vi "Send.vi"(6 "Timeout":T1={"mode"=enum."Relative", "deadline (ms)"=30000}, 7 "priority":bool, 8 "error in (no error)":errorcluster, 9 "path":string, 10 "session in":refnum<class "Session.lvclass">, 11 "NI_SFTP.lvlib:statvfs_openssh.com.lvclass":refnum<class "statvfs_openssh.com.lvclass">) -> (0 "error out":errorcluster, 1 "request id":u32, 2 "session out":refnum<class "Session.lvclass">, 3 "NI_SFTP.lvlib:statvfs_openssh.com.lvclass 2":refnum<class "statvfs_openssh.com.lvclass">)   [LabVIEW 2020, in "NI_SFTP.lvlib" / "statvfs_openssh.com.lvclass"]
uses:
  <vilib>/net/SFTP/API/Support/Command/statvfs_openssh.com/statvfs_openssh.com.lvclass
  <vilib>/net/SFTP/Session/Session.lvclass
  <vilib>/Utility/Deadline/Deadline.ctl
  <vilib>/Utility/Deadline/Mode.ctl
  <vilib>/net/SFTP/API/Support/Command/SSH_FXP_EXTENDED/Input.ctl
  <vilib>/net/SFTP/Low Level Connection/Serialize Byte Array.vi
  <vilib>/net/SFTP/API/Support/Command/SSH_FXP_EXTENDED/SSH_FXP_EXTENDED.lvclass
  <vilib>/net/SFTP/NI_SFTP.lvlib
  <vilib>/net/SFTP/Low Level Connection/Low Level Connection.lvclass
  <vilib>/Utility/Deadline/NI_Deadline.lvlib
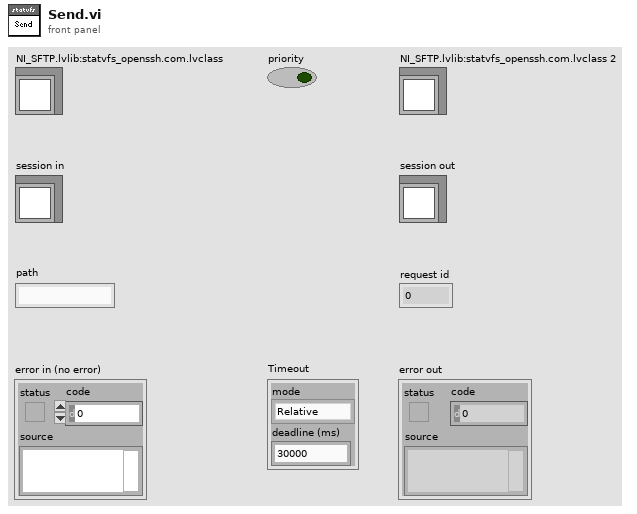
[diagram p1: front panel]
types:
  T1 = typedef "NI_Deadline.lvlib/Deadline.ctl" = cluster{"mode":T2, "deadline (ms)":u32}
  T2 = typedef "NI_Deadline.lvlib/Mode.ctl" = enum16{"Relative", "Use deadline", "Wait forever", "Nonblocking", "N/A"}
  T3 = typedef "NI_SFTP.lvlib/SSH_FXP_EXTENDED.lvclass/Input.ctl" = cluster{"extended-request":string, "payload":u8[]}
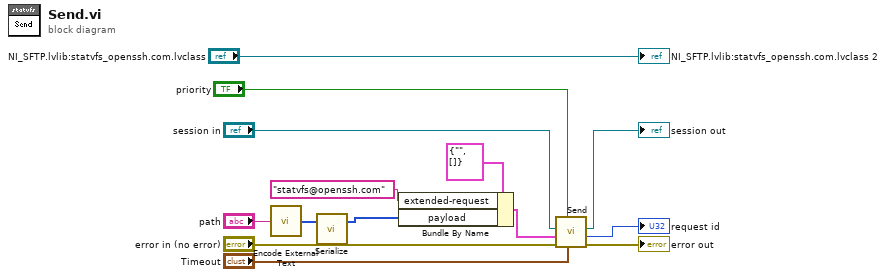
[diagram p0: block diagram]
diagram:
  n1 = call <vilib>:"Encode External Text.vi"("string"="path") -> ("data"=w10:u8[])
  n2 = call-poly <vilib>:"Serialize.vi"("data"=w10) -> ("bytes"=w8:u8[])  [unwired: 2 in]
  n3 = Bundle By Name(cluster=T3 {"extended-request"="", "payload"=[]} ("input"), "extended-request"="statvfs@openssh.com", "payload"=w8) -> (w6:T3)
  n4 = call <vilib>:"Send.vi"("Timeout"="Timeout", "priority"="priority", "error in"="error in (no error)", "input"=w6, "session in"="session in") -> ("error out"=→"error out":errorcluster, "request id"=→"request id":u32, "session out"=→"session out":refnum<class "Session.lvclass">)  [unwired: 3 in, 1 out]
  "NI_SFTP.lvlib:statvfs_openssh.com.lvclass 2" <- "NI_SFTP.lvlib:statvfs_openssh.com.lvclass"
